vi "Write Units.vi"(8 "error in (no error)":errorcluster, 10 "Units":T1, 11 "Units in":refnum<class "Units.lvclass">) -> (0 "error out":errorcluster, 3 "Units out":refnum<class "Units.lvclass">)   [LabVIEW 2013, in "MaterialCharacterization.lvlib" / "Units.lvclass"]
uses:
  Units.lvclass
  ScanParser/Units.ctl
  Units.lvclass/Units.ctl
  ScanParser/MC-ScanParser.lvclass
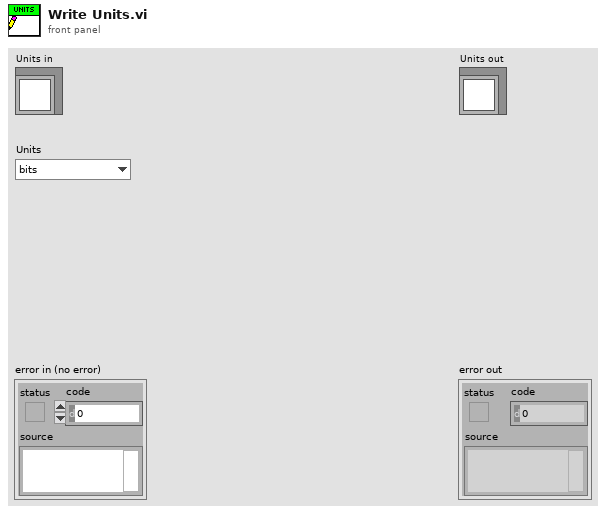
[diagram p1: front panel]
types:
  T1 = typedef "MaterialCharacterization.lvlib/MC-ScanParser.lvclass/Units.ctl" = enum16{"bits", "mm", "inch", "mils"}
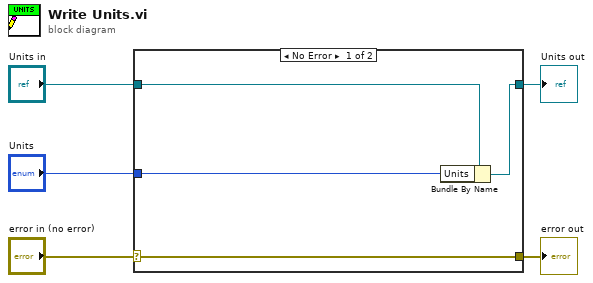
[diagram p0: block diagram]
diagram:
  n1 = case shown="No Error" "error in (no error)" {
    selector: "error in (no error)" -> [w9 w10]
    tunnel: [w9 w10] -> w4
    tunnel: [w7 w11] -> w2
    tunnel: "Units in" -> [w8 w11]
    tunnel: "Units" -> [w6 _]
    frame No Error {
      n2 = Bundle By Name(cluster=w8, "Units"=w6) -> (w7:refnum<class "Units.lvclass">)
    }
    frame Error {
    }
  }
  "error out" <- w4
  "Units out" <- w2
